vi "Milliseconds To Wait From Global.vi"(8 "error in (no error)":errorcluster, 11 "milliseconds to wait":u32) -> (0 "error out":errorcluster)   [LabVIEW 2015]
doc: "Waits the specified number of miliseconds."
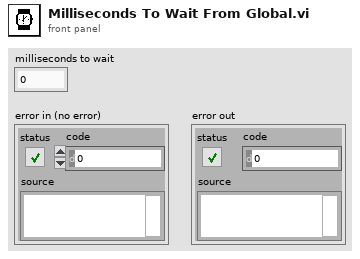
[diagram p1: front panel]
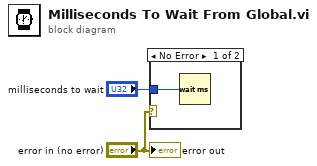
[diagram p0: block diagram]
diagram:
  n1 = case shown="No Error" "error in (no error)" {
    tunnel: "milliseconds to wait" -> [w3 _]
    frame No Error {
      n2 = Wait (ms)(milliseconds to wait=w3) -> ()  [unwired: 1 out]
    }
    frame Error {
    }
  }
  "error out" <- "error in (no error)"
